vi "LVCAM Destroy.vi"(10 "Error":errorcluster, 11 "Process in":refnum<class "Process.lvclass">) -> ()   [LabVIEW 2021, in "Process.lvlib" / "Process.lvclass"]
uses:
  Process.lvclass
  Process.lvclass/Process.ctl
  LVCAM/LVCAM/LVCAM/LVCAM.lvclass
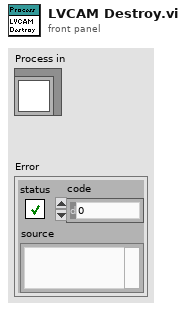
[diagram p1: front panel]
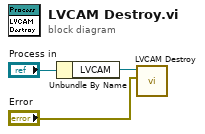
[diagram p0: block diagram]
diagram:
  n1 = Unbundle By Name("Process in") -> ("LVCAM"=w2:refnum<class "LVCAM.lvclass">)
  n2 = call-dynamic "LVCAM Destroy.vi"("Error"="Error", "LVCAM Destroy in"=w2) -> ()  [unwired: 10 in]
